vi "DC_run.vi"(0 "KNR in":T2, 1 "speed_1":dbl format="%.2f", 2 "reinitialize? (F)":bool, 3 "error in (no error)":errorcluster, 5 "speed_2":dbl format="%.2f") -> (4 "Position_1":i32, 6 "KNR out":T2, 8 "Position_2":i32, 9 "error out":errorcluster)   [LabVIEW 2013]
uses:
  <userlib>/KNR OS 3.0 LabVIEW Toolkit/Type Definition/KNR3 Reference.ctl
  <userlib>/_FPGA Interface Advanced Tools/FPGA Interface Base/FPGA Interface Base.lvclass
  <userlib>/KNR OS 3.0 LabVIEW Toolkit/Type Definition/Resource.ctl
  Global 1.vi
  <vilib>/addons/control/pid/pid.llb/PID (DBL).vi
  <vilib>/addons/control/pid/NI_PID_pid.lvlib
panel:
  out "Pos":T1(graph)
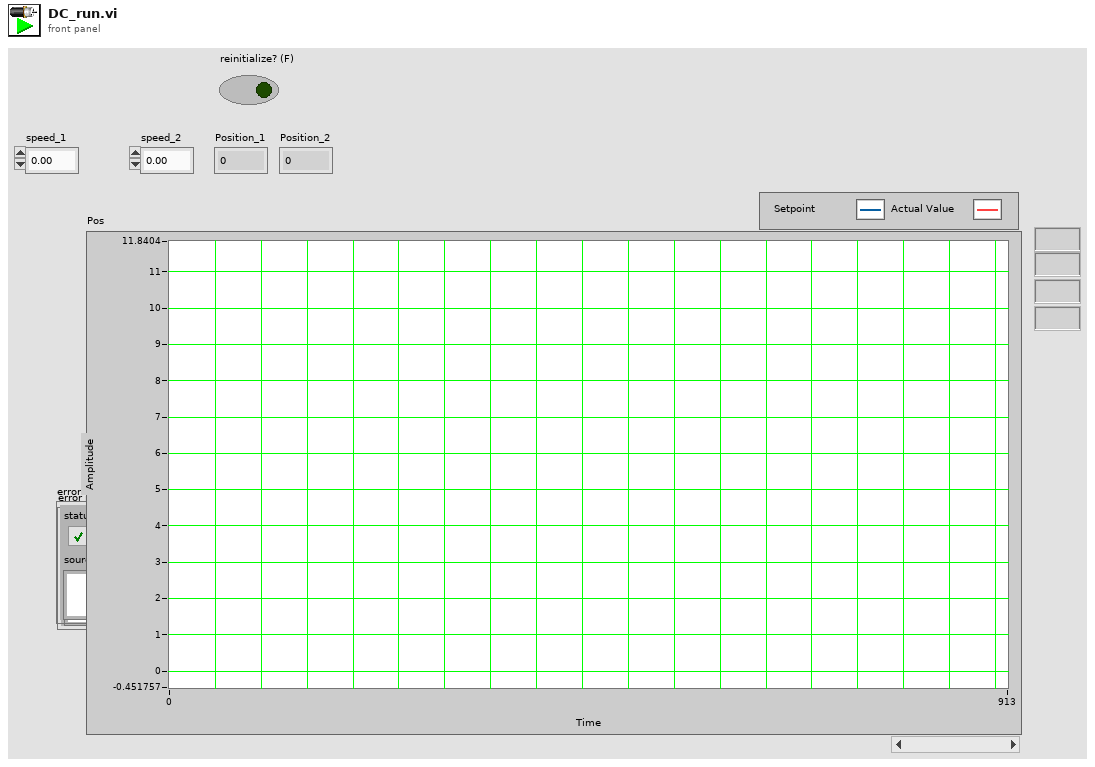
[diagram p1: front panel]
types:
  T1 = cluster{"CM":dbl, "speed_2":dbl, "CM":dbl, "speed_1":dbl}
  T2 = typedef "KNR3 Reference.ctl" = cluster{"FPGA Session":refnum<class "FPGA Interface Base.lvclass">, "Resource":T3}
  T3 = typedef "Resource.ctl" = enum16{"KNRm_DDRC", "KNRm_DDDD", "KNRm_DDDR", "KNRm_DDDC", "KNR"}
  T4 = cluster{"proportional gain (Kc)":dbl, "integral time (Ti, min)":dbl, "derivative time (Td, min)":dbl}
  T5 = typedef "DC Motor Port.ctl" = u16
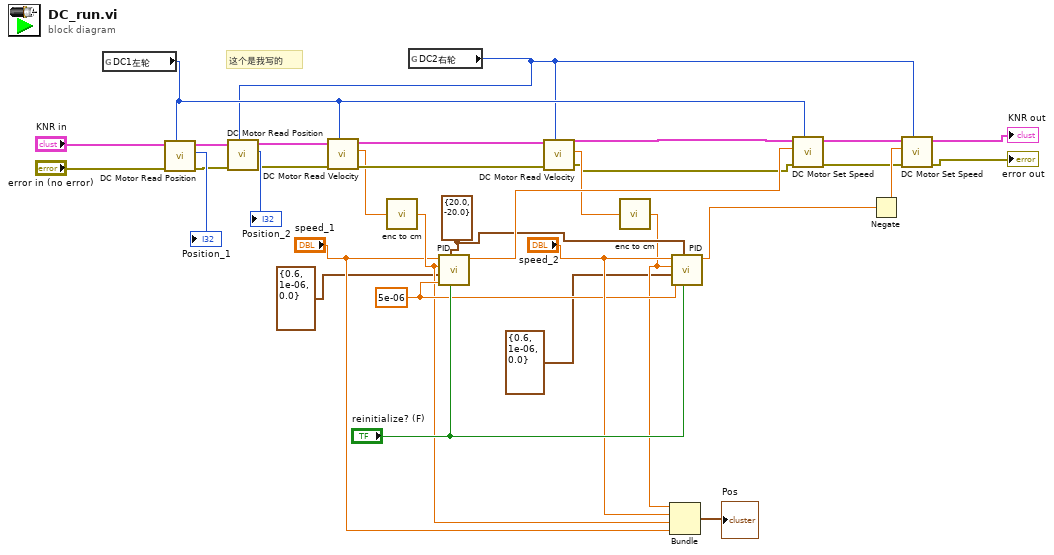
[diagram p0: block diagram]
diagram:
  w7 = cluster{"output high":dbl, "output low":dbl} {"output high"=20.0, "output low"=-20.0} ("output range")
  w8 = 5e-06 ("dt (s)")
  # "这个是我写的"
  n1 = global read "Global 1.vi" "DC1左轮"() -> (w10:T5)
  n2 = call <userlib>:"DC Motor Read Position.vi"("Port (DS1)"=w10, "error in (no error)"="error in (no error)", "KNR in"="KNR in") -> ("error out"=w29:errorcluster, "Position"=→"Position_1":i32, "KNR out"=w26:T2)  [unwired: 6 in]
  n3 = global read "Global 1.vi" "DC2右轮"() -> (w9:T5)
  n4 = call <userlib>:"DC Motor Read Position.vi"("Port (DS1)"=w9, "error in (no error)"=w29, "KNR in"=w26) -> ("error out"=w28:errorcluster, "Position"=→"Position_2":i32, "KNR out"=w27:T2)  [unwired: 6 in]
  n5 = call <userlib>:"DC Motor Read Velocity.vi"("Port (DS1)"=w10, "error in (no error)"=w28, "KNR in"=w27) -> ("error out"=w22:errorcluster, "Velocity (cts/sec)"=w19:dbl, "KNR out"=w21:T2)  [unwired: 6 in]
  n6 = call "enc to cm.vi"("E"=w19) -> ("CM"=w4:dbl)  [unwired: 1 in]
  n7 = call-poly <vilib>:"PID.vi"("reinitialize? (F)"="reinitialize? (F)", "output range"=w7, "dt (s)"=w8, "PID gains"=T4 {"proportional gain (Kc)"=0.6, "integral time (Ti, min)"=1e-06, "derivative time (Td, min)"=0.0}, "process variable"=w4, "setpoint"="speed_1") -> ("output"=w25:dbl)  [unwired: 4 in, 1 out]
  n8 = call <userlib>:"DC Motor Read Velocity.vi"("Port (DS1)"=w9, "error in (no error)"=w22, "KNR in"=w21) -> ("error out"=w11:errorcluster, "Velocity (cts/sec)"=w20:dbl, "KNR out"=w12:T2)  [unwired: 6 in]
  n9 = call "enc to cm.vi"("E"=w20) -> ("CM"=w5:dbl)  [unwired: 1 in]
  n10 = Bundle("CM"=w5, "speed_2"="speed_2", "CM"=w4, "speed_1"="speed_1") -> (→"Pos":T1)  [unwired: 1 in]
  n11 = call-poly <vilib>:"PID.vi"("reinitialize? (F)"="reinitialize? (F)", "output range"=w7, "dt (s)"=w8, "PID gains"=T4 {"proportional gain (Kc)"=0.6, "integral time (Ti, min)"=1e-06, "derivative time (Td, min)"=0.0}, "process variable"=w5, "setpoint"="speed_2") -> ("output"=w24:dbl)  [unwired: 4 in, 1 out]
  n12 = call <userlib>:"DC Motor Set Speed.vi"("Port (DS1)"=w10, "error in (no error)"=w11, "Speed (+-100%)"=w25, "KNR in"=w12) -> ("error out"=w13:errorcluster, "KNR out"=w14:T2)  [unwired: 6 in]
  n13 = Negate(x=w24) -> (-x=w23:dbl)
  n14 = call <userlib>:"DC Motor Set Speed.vi"("Port (DS1)"=w9, "error in (no error)"=w13, "Speed (+-100%)"=w23, "KNR in"=w14) -> ("error out"=→"error out":errorcluster, "KNR out"=→"KNR out":T2)  [unwired: 6 in]
